vi "Mixer.Enqueue Action.vi"(0 "action":string, 7 "data":variant, 11 "error in (no error)":errorcluster) -> (15 "error out":errorcluster)   [LabVIEW 2020]
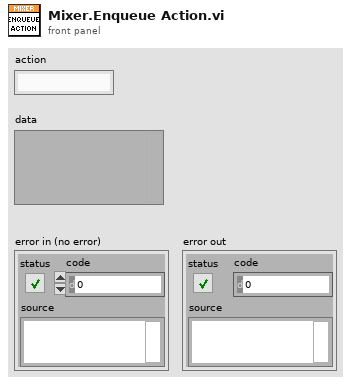
[diagram p1: front panel]
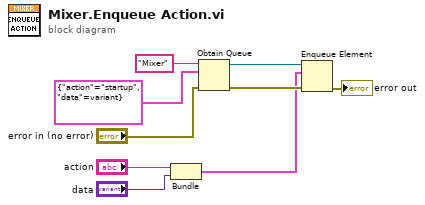
[diagram p0: block diagram]
diagram:
  n1 = Bundle("action"="action", "data"="data") -> (w2:cluster{"action":string, "data":variant})  [unwired: 1 in]
  n2 = Obtain Queue(name (unnamed)="Mixer", element data type=cluster{"action":string, "data":variant} {"action"="startup", "data"=variant}, error in (no error)="error in (no error)") -> (queue out=w8:refnum<queue>, error out=w5:errorcluster)  [unwired: 2 in, 1 out]
  n3 = Enqueue Element(queue=w8, element=w2, error in (no error)=w5) -> (error out=→"error out":errorcluster)  [unwired: 1 in, 2 out]
